vi "File.Path, Resolve Path Variables.vi"(10 "Variables":string[][](array[string])=[["$Date", ""], ["$Year", ""], ["$Month", ""], ["$Day", ""]], 11 "Path":path) -> (2 "Variables Out":string[][](array[string])=[["$Date", ""], ["$Year", ""], ["$Month", ""], ["$Day", ""]], 3 "Path Out":path)   [LabVIEW 2019]
panel:
  out "Changed":bool
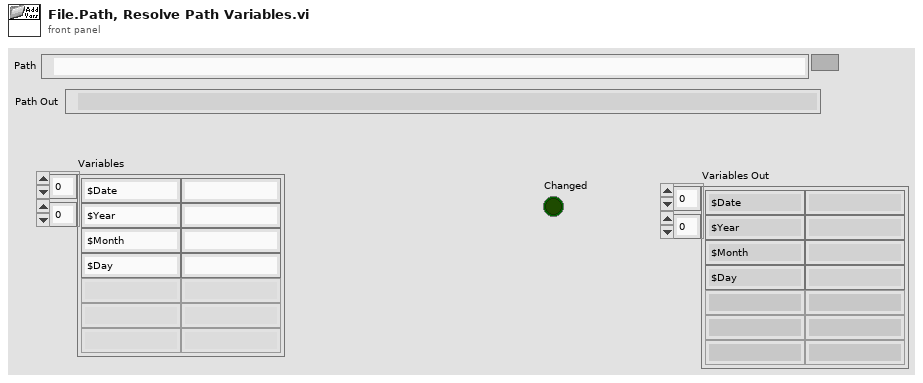
[diagram p1: front panel]
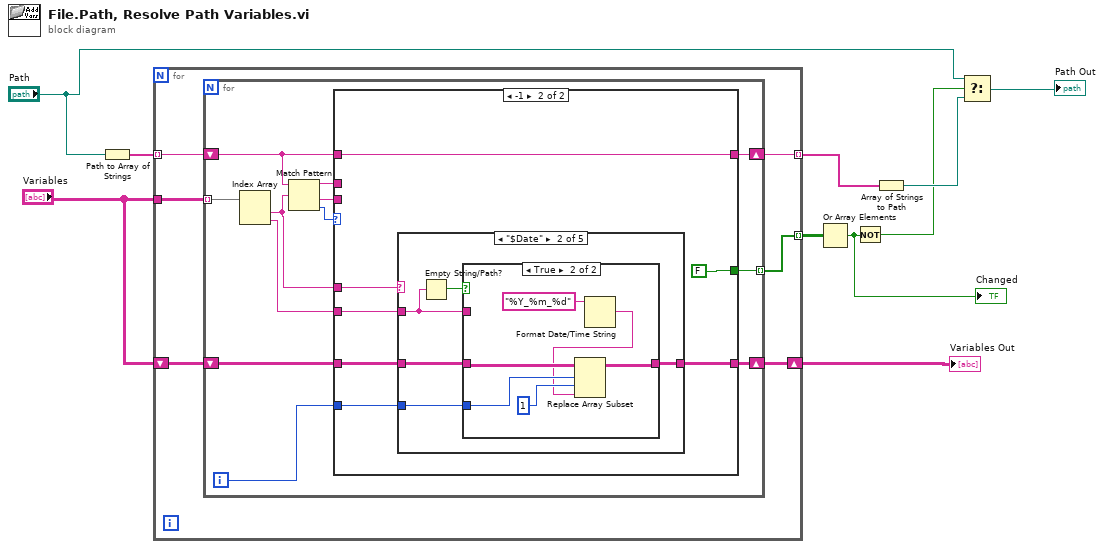
[diagram p0: block diagram]
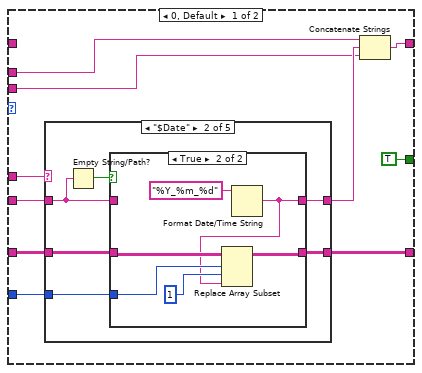
[diagram p2: hidden frame]
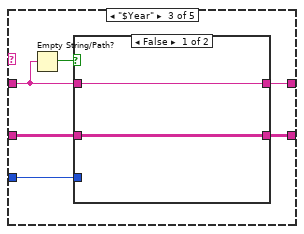
[diagram p5: hidden frame]
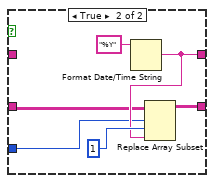
[diagram p6: hidden frame]
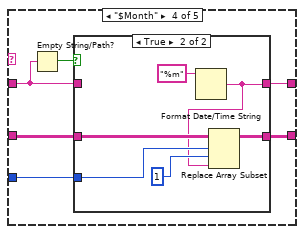
[diagram p7: hidden frame]
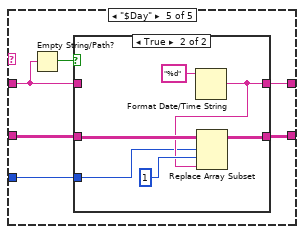
[diagram p9: hidden frame]
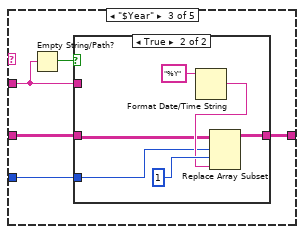
[diagram p13: hidden frame]
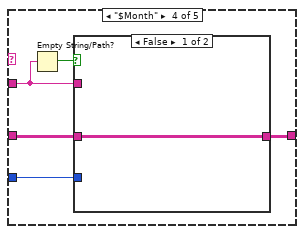
[diagram p15: hidden frame]
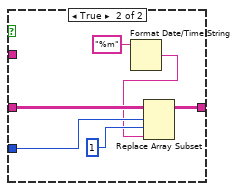
[diagram p16: hidden frame]
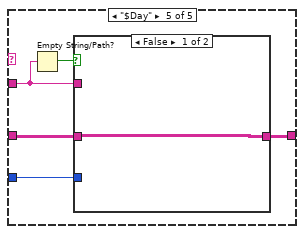
[diagram p17: hidden frame]
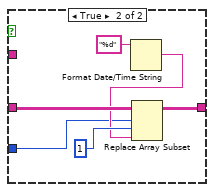
[diagram p18: hidden frame]
diagram:
  n1 = Path to Array of Strings(0:"Path") -> (2:w10:string[])  [unwired: 1 out]
  n2 = for {
    tunnel: w10 -> [w15] mode=indexing
    tunnel: "Variables" -> [w16]
    tunnel: [w14] -> w6 mode=indexing
    tunnel: [w13] -> w5 mode=indexing
    shift-right: [w11] -> w1
    shift-left: "Variables" -> [w12]
    n3 = for {
      tunnel: w16 -> [w28] mode=indexing
      shift-right: [w22] -> w13
      shift-left: w15 -> [w23]
      tunnel: [w21] -> w14 mode=indexing
      shift-right: [w18] -> w11
      shift-left: w12 -> [w19]
      i -> [w17]
      n4 = Index Array(array=w28) -> (element #1=w20:string, element #2=w24:string)  [unwired: 2 in]
      n5 = Match Pattern(string=w23, regular expression=w20) -> (before substring=w26:string, after substring=w25:string, offset past match=w27:i32)  [unwired: 1 in, 1 out]
      n6 = case shown="-1" w27 {
        tunnel: w26 -> [w35 _]
        tunnel: w25 -> [w33 _]
        tunnel: w24 -> [w37 w100]
        tunnel: w23 -> [_ w103]
        tunnel: [w36 w103] -> w22
        tunnel: [TRUE FALSE] -> w21
        tunnel: w20 -> [w38 w101]
        tunnel: w19 -> [w31 w99]
        tunnel: [w30 w97] -> w18
        tunnel: w17 -> [w29 w98]
        frame 0, Default {
          n7 = case shown="\"$Date\"" w38 {
            tunnel: w37 -> [w40 w45 w59 w73 w87]
            tunnel: [w40 w44 w58 w72 w86] -> w34
            tunnel: w31 -> [w39 w43 w57 w71 w84]
            tunnel: [w39 w42 w56 w70 w85] -> w30
            tunnel: w29 -> [_ w41 w55 w69 w83]
            frame Default {
            }
            frame "$Date" {
              n8 = Empty String/Path?(string/path=w45) -> (empty?=w46:bool)
              n9 = case shown="True" w46 {
                tunnel: w45 -> [w48 _]
                tunnel: [w48 w50] -> w44
                tunnel: w43 -> [w47 w52]
                tunnel: [w47 w49] -> w42
                tunnel: w41 -> [_ w51]
                frame False {
                }
                frame True {
                  n10 = Format Date/Time String(time format string (%c)="%Y_%m_%d") -> (date/time string=w50:string)  [unwired: 2 in]
                  n11 = Replace Array Subset(array=w52, new element=w50, index (row)=w51, index (col)=1 ("disabled index (col)")) -> (w49:string[][])
                }
              }
            }
            frame "$Year" {
              n12 = Empty String/Path?(string/path=w59) -> (empty?=w60:bool)
              n13 = case shown="False" w60 {
                tunnel: w59 -> [w62 _]
                tunnel: [w62 w65] -> w58
                tunnel: w57 -> [w61 w64]
                tunnel: [w61 w66] -> w56
                tunnel: w55 -> [_ w63]
                frame False {
                }
                frame True {
                  n14 = Format Date/Time String(time format string (%c)="%Y") -> (date/time string=w65:string)  [unwired: 2 in]
                  n15 = Replace Array Subset(array=w64, new element=w65, index (row)=w63, index (col)=1 ("disabled index (col)")) -> (w66:string[][])
                }
              }
            }
            frame "$Month" {
              n16 = Empty String/Path?(string/path=w73) -> (empty?=w74:bool)
              n17 = case shown="True" w74 {
                tunnel: w73 -> [w75 _]
                tunnel: [w75 w77] -> w72
                tunnel: w71 -> [w76 w79]
                tunnel: [w76 w80] -> w70
                tunnel: w69 -> [_ w78]
                frame False {
                }
                frame True {
                  n18 = Format Date/Time String(time format string (%c)="%m") -> (date/time string=w77:string)  [unwired: 2 in]
                  n19 = Replace Array Subset(array=w79, new element=w77, index (row)=w78, index (col)=1 ("disabled index (col)")) -> (w80:string[][])
                }
              }
            }
            frame "$Day" {
              n20 = Empty String/Path?(string/path=w87) -> (empty?=w88:bool)
              n21 = case shown="True" w88 {
                tunnel: w87 -> [w90 _]
                tunnel: [w90 w92] -> w86
                tunnel: [w89 w94] -> w85
                tunnel: w84 -> [w89 w93]
                tunnel: w83 -> [_ w91]
                frame False {
                }
                frame True {
                  n22 = Format Date/Time String(time format string (%c)="%d") -> (date/time string=w92:string)  [unwired: 2 in]
                  n23 = Replace Array Subset(array=w93, new element=w92, index (row)=w91, index (col)=1 ("disabled index (col)")) -> (w94:string[][])
                }
              }
            }
          }
          n24 = Concatenate Strings(w35, w34, w33) -> (w36:string)
        }
        frame -1 {
          n25 = case shown="\"$Date\"" w101 {
            tunnel: w100 -> [_ w108 w120 w132 w144]
            tunnel: w99 -> [w104 w107 w119 w131 w142]
            tunnel: [w104 w106 w118 w130 w143] -> w97
            tunnel: w98 -> [_ w105 w117 w129 w141]
            frame Default {
            }
            frame "$Date" {
              n26 = Empty String/Path?(string/path=w108) -> (empty?=w109:bool)
              n27 = case shown="True" w109 {
                tunnel: w108 -> [_ _]
                tunnel: w107 -> [w110 w114]
                tunnel: [w110 w111] -> w106
                tunnel: w105 -> [_ w113]
                frame False {
                }
                frame True {
                  n28 = Format Date/Time String(time format string (%c)="%Y_%m_%d") -> (date/time string=w112:string)  [unwired: 2 in]
                  n29 = Replace Array Subset(array=w114, new element=w112, index (row)=w113, index (col)=1 ("disabled index (col)")) -> (w111:string[][])
                }
              }
            }
            frame "$Year" {
              n30 = Empty String/Path?(string/path=w120) -> (empty?=w121:bool)
              n31 = case shown="True" w121 {
                tunnel: w120 -> [_ _]
                tunnel: w119 -> [w122 w124]
                tunnel: [w122 w126] -> w118
                tunnel: w117 -> [_ w123]
                frame False {
                }
                frame True {
                  n32 = Format Date/Time String(time format string (%c)="%Y") -> (date/time string=w125:string)  [unwired: 2 in]
                  n33 = Replace Array Subset(array=w124, new element=w125, index (row)=w123, index (col)=1 ("disabled index (col)")) -> (w126:string[][])
                }
              }
            }
            frame "$Month" {
              n34 = Empty String/Path?(string/path=w132) -> (empty?=w133:bool)
              n35 = case shown="False" w133 {
                tunnel: w132 -> [_ _]
                tunnel: w131 -> [w134 w137]
                tunnel: [w134 w138] -> w130
                tunnel: w129 -> [_ w136]
                frame False {
                }
                frame True {
                  n36 = Format Date/Time String(time format string (%c)="%m") -> (date/time string=w135:string)  [unwired: 2 in]
                  n37 = Replace Array Subset(array=w137, new element=w135, index (row)=w136, index (col)=1 ("disabled index (col)")) -> (w138:string[][])
                }
              }
            }
            frame "$Day" {
              n38 = Empty String/Path?(string/path=w144) -> (empty?=w145:bool)
              n39 = case shown="False" w145 {
                tunnel: w144 -> [_ _]
                tunnel: [w146 w150] -> w143
                tunnel: w142 -> [w146 w149]
                tunnel: w141 -> [_ w147]
                frame False {
                }
                frame True {
                  n40 = Format Date/Time String(time format string (%c)="%d") -> (date/time string=w148:string)  [unwired: 2 in]
                  n41 = Replace Array Subset(array=w149, new element=w148, index (row)=w147, index (col)=1 ("disabled index (col)")) -> (w150:string[][])
                }
              }
            }
          }
        }
      }
    }
  }
  "Variables Out" <- w1
  n42 = Or Array Elements(Boolean array=w6) -> (logical OR=w3:bool)
  "Changed" <- w3
  n43 = Not(x=w3) -> (.not. x?=w4:bool)
  n44 = Array of Strings to Path(0:w5) -> (2:w7:path)  [unwired: 1 in]
  n45 = Select(t="Path", s=w4, f=w7) -> (s? t:f=→"Path Out":path)
